vi "test_response string.vi"(8 "error in (no error)":errorcluster, 11 "TestCase in":refnum<class "Return Response Triggers.lvclass">) -> (0 "error out":errorcluster, 3 "TestCase out":refnum<class "Return Response Triggers.lvclass">)   [LabVIEW 2017, in "SSH.lvlib" / "Return Response Triggers.lvclass"]
uses:
  Return Response Triggers.lvclass
  Return Request Configuration.ctl
  Response Configuration.ctl
  <vilib>/addons/_JKI Toolkits/VI Tester/TestCase.llb/TestCase.lvclass
  SSH.lvlib
  C:/Program Files (x86)/National Instruments/LabVIEW 2017/vi.lib/addons/_JKI Toolkits/VI Tester/TestCase.llb/TestCase.lvclass
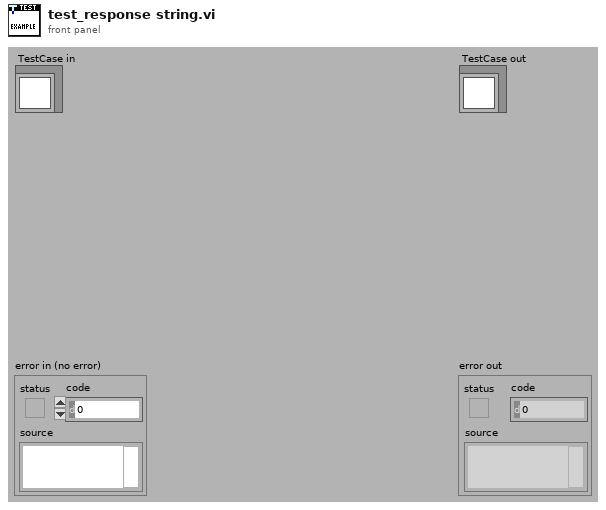
[diagram p1: front panel]
types:
  T1 = typedef "SSH.lvlib/Return Request Configuration.ctl" = cluster{"Response Configuration":T2, "Return Notifier":refnum<notifier>, "Response Requested":bool, "Command":string, "Initial Timer Value":u32}
  T2 = typedef "SSH.lvlib/Response Configuration.ctl" = cluster{"Expected Response":string, "Character Count Limit":i32, "Timeout (ms)":u32}
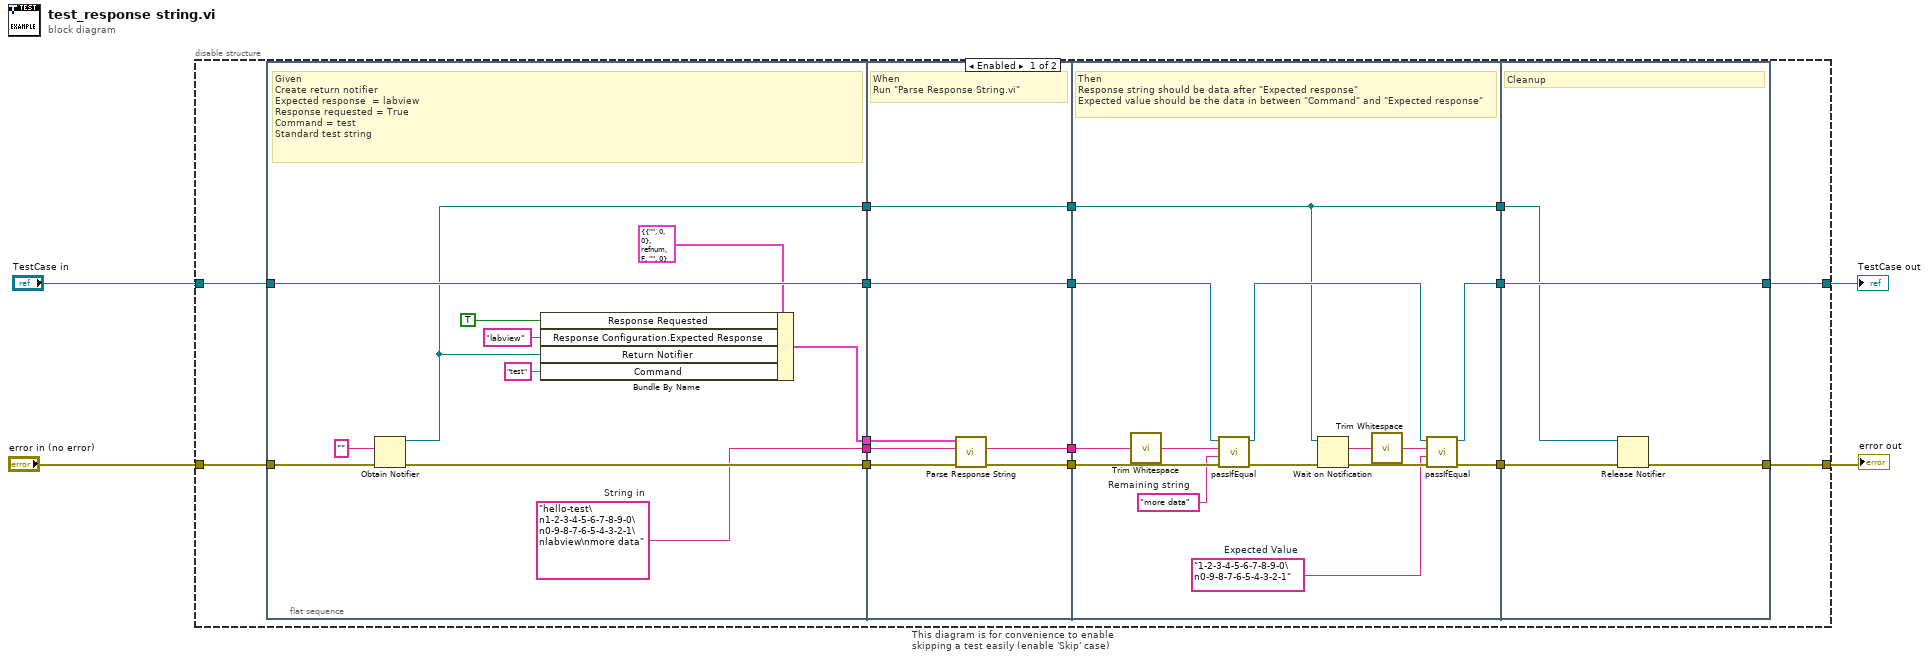
[diagram p0: block diagram]
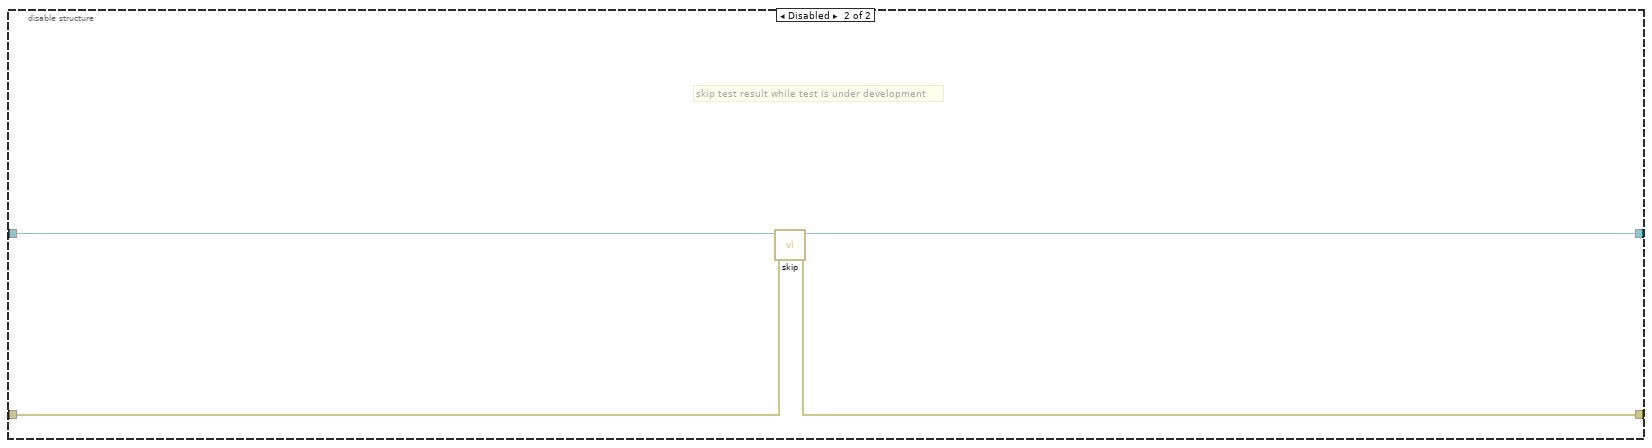
[diagram p2: hidden frame]
diagram:
  n1 = disable-structure "This diagram is for convenience to enable skipping a test easily (enable 'Skip' case)" shown="Enabled" {
    disable-tunnel: "TestCase in" -> [w13 w60]
    disable-tunnel: [w12 w58] -> w1
    disable-tunnel: [w11 w59] -> w3
    disable-tunnel: "error in (no error)" -> [w14 w57]
    frame Enabled {
      n2 = flat-sequence {
        tunnel: w14 -> [w28]
        tunnel: w13 -> [w31]
        tunnel: [w31] -> w20
        tunnel: [w27] -> w19
        tunnel: [w26] -> w10
        tunnel: [w22] -> w9
        tunnel: [w21] -> w8
        tunnel: [w38] -> w18
        tunnel: [w36] -> w17
        tunnel: w20 -> [w38]
        tunnel: w19 -> [w37]
        tunnel: w10 -> [w35]
        tunnel: w9 -> [w32]
        tunnel: w8 -> [w34]
        tunnel: [w33] -> w7
        tunnel: [w32] -> w6
        tunnel: [w45] -> w16
        tunnel: [w47] -> w15
        tunnel: w18 -> [w52]
        tunnel: w17 -> [w51]
        tunnel: w7 -> [w49]
        tunnel: w6 -> [w42]
        tunnel: [w42] -> w5
        tunnel: [w54] -> w11
        tunnel: [w56] -> w12
        tunnel: w16 -> [w56]
        tunnel: w15 -> [w55]
        tunnel: w5 -> [w53]
        frame #0 {
          w21 = "hello-test\n1-2-3-4-5-6-7-8-9-0\n0-9-8-7-6-5-4-3-2-1\nlabview\nmore data"  # String in
          # "Given\nCreate return notifier\nExpected response  = labview\nResponse requested = True\nCommand = test\nStandard test string"
          n3 = Obtain Notifier(notification data type="", error in (no error)=w28) -> (notifier out=w22:refnum<notifier>, error out=w27:errorcluster)  [unwired: 2 in, 1 out]
          n4 = Bundle By Name(cluster=T1 {"Response Configuration"={"Expected Response"="", "Character Count Limit"=0, "Timeout (ms)"=0}, "Return Notifier"=refnum, "Response Requested"=FALSE, "Command"="", "Initial Timer Value"=0} ("Return Request in"), "Response Requested"=TRUE, "Response Configuration.Expected Response"="labview", "Return Notifier"=w22, "Command"="test") -> (w26:T1)
        }
        frame #1 {
          # "When\nRun \"Parse Response String.vi\""
          n5 = call "Parse Response String.vi"("error in (no error)"=w37, "Response String in"=w34, "Return Request in"=w35) -> ("error out"=w36:errorcluster, "Response String out"=w33:string)  [unwired: 6 in, 1 out]
        }
        frame #2 {
          w41 = "more data"  # Remaining string
          w44 = "1-2-3-4-5-6-7-8-9-0\n0-9-8-7-6-5-4-3-2-1"  # Expected Value
          # "Then\nResponse string should be data after \"Expected response\"\nExpected value should be the data in between \"Command\" and \"Expected response\""
          n6 = call <vilib>:"Trim Whitespace.vi"("string"=w49) -> ("trimmed string"=w40:string)  [unwired: 1 in]
          n7 = call-dynamic "passIfEqual.vi"("error in (no error)"=w51, "y"=w41, "x"=w40, "TestCase in"=w52) -> ("error out"=w50:errorcluster, "TestCase out"=w46:refnum<class "Return Response Triggers.lvclass">)  [unwired: 6 in]
          n8 = Wait on Notification(notifier=w42, error in (no error)=w50) -> (notification=w43:string, error out=w48:errorcluster)  [unwired: 2 in, 2 out]
          n9 = call <vilib>:"Trim Whitespace.vi"("string"=w43) -> ("trimmed string"=w39:string)  [unwired: 1 in]
          n10 = call-dynamic "passIfEqual.vi"("error in (no error)"=w48, "y"=w44, "x"=w39, "TestCase in"=w46) -> ("error out"=w47:errorcluster, "TestCase out"=w45:refnum<class "Return Response Triggers.lvclass">)  [unwired: 6 in]
        }
        frame #3 {
          # "Cleanup"
          n11 = Release Notifier(notifier=w53, error in (no error)=w55) -> (error out=w54:errorcluster)  [unwired: 1 in, 2 out]
        }
      }
    }
    frame Disabled {
      # "skip test result while test is under development"
      n12 = call <vilib>:"skip.vi"("error in (no error)"=w57, "TestCase in"=w60) -> ("error out"=w59:errorcluster, "TestCase out"=w58:refnum<class "Return Response Triggers.lvclass">)  [unwired: 8 in]
    }
  }
  "error out" <- w3
  "TestCase out" <- w1
